vi "Degrees_To_Encoder.vi"(8 "Max Encoder Value":dbl=0.58904, 9 "Degrees Rotation":dbl=250.0, 11 "Degree Value":dbl) -> (3 "Encoder Value":dbl)   [LabVIEW 2012]
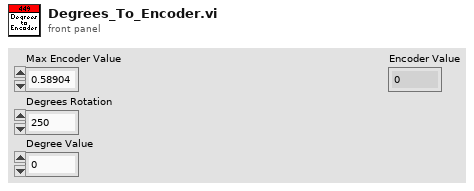
[diagram p1: front panel]
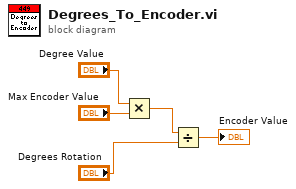
[diagram p0: block diagram]
diagram:
  n1 = Multiply(x="Degree Value", y="Max Encoder Value") -> (x*y=w5:dbl)
  n2 = Divide(x=w5, y="Degrees Rotation") -> (x/y=→"Encoder Value":dbl)
